vi "Get Item Reference By PathName.vi"(8 "error in (no error)":errorcluster, 10 "Item PathName":string, 11 "Root Item Reference in":T1 format="%.0x") -> (0 "error out":errorcluster, 2 "Item Reference":u64 format="%.0x", 3 "Root Item Reference out":T1 format="%.0x", 4 "found":bool)   [LabVIEW 2013, in "Hierarchy Framework.lvlib" / "Item.lvclass"]
uses:
  Item.lvclass
  Ctls/Item Reference.ctl
  Section/Section.lvclass
  Generic/Generic.lvclass
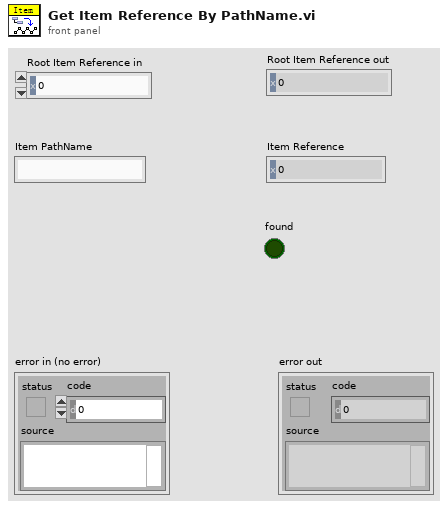
[diagram p1: front panel]
types:
  T1 = typedef "Hierarchy Framework.lvlib/Item.lvclass/Item Reference.ctl" = u64
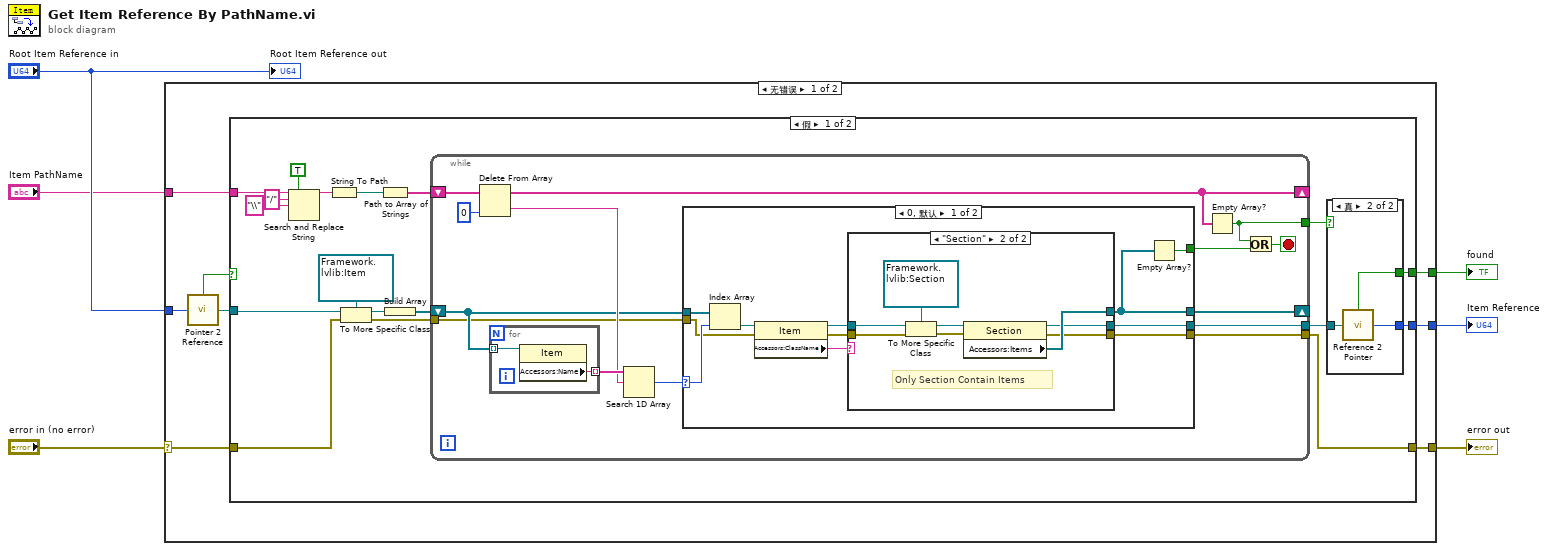
[diagram p0: block diagram]
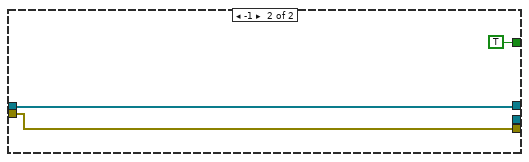
[diagram p4: hidden frame]
diagram:
  n1 = case shown="无错误" "error in (no error)" {
    selector: "error in (no error)" -> [w13 w77]
    tunnel: "Root Item Reference in" -> [w12 _]
    tunnel: [w14 w77] -> w5
    tunnel: [w9 _] -> w3
    tunnel: "Item PathName" -> [w8 _]
    tunnel: [w7 _] -> w1
    frame No Error {
      n2 = call "Pointer 2 Reference.vi"("Pointer"=w12) -> ("Not A Refnum?"=w11:bool, "Generic Reference"=w10:refnum<data-value>)
      n3 = case shown="假" w11 {
        tunnel: w13 -> [w31 w76]
        tunnel: [w25 w76] -> w14
        tunnel: w10 -> [w32 _]
        tunnel: [w16 _] -> w9
        tunnel: w8 -> [w22 _]
        tunnel: [w24 _] -> w7
        frame False {
          n4 = Search and Replace String(replace all?=TRUE ("替换全部？(F)"), input string=w22, search string="/" ("搜索字符串"), replace string="\\" ("替换字符串(\"\")")) -> (result string=w21:string)  [unwired: 4 in, 3 out]
          n5 = String To Path(string=w21) -> (path=w23:path)
          n6 = To More Specific Class(target class=refnum<data-value> refnum ("Item"), reference=w32, error in=w31) -> (specific class reference=w27:refnum<data-value>, error out=w26:errorcluster)
          n7 = Path to Array of Strings(0:w23) -> (2:w28:string[])  [unwired: 1 out]
          n8 = Build Array(w27) -> (w29:refnum<data-value>[])
          n9 = while {
            shift-right: [w45] -> _
            shift-left: w28 -> [w49]
            shift-right: [w41] -> _
            shift-left: w29 -> [w42]
            tunnel: [w40] -> w17
            tunnel: [w39] -> w25
            tunnel: w26 -> [w38]
            tunnel: [w36] -> w15
            stop <- w44 stop-if-true
            n10 = Delete From Array(array=w49, index=0 ("索引")) -> (deleted portion=w46:string, array with subset deleted=w45:string[])  [unwired: 1 in]
            n11 = for {
              tunnel: w42 -> [w75] mode=indexing
              tunnel: [w74] -> w47 mode=indexing
              n12 = property class="Item"(reference=w75) -> ("Accessors:Name"=w74:string)  [unwired: 1 in, 2 out]
            }
            n13 = Search 1D Array(1D array=w47, element=w46) -> (index of element=w43:i32)  [unwired: 1 in]
            n14 = case shown="0, 默认" w43 {
              selector: w43 -> [w59 _]
              tunnel: w42 -> [w60 w73]
              tunnel: [w50 w73] -> w41
              tunnel: [w54 _] -> w40
              tunnel: [w53 w72] -> w39
              tunnel: w38 -> [w52 w72]
              tunnel: [w51 TRUE] -> w37
              frame 0, Default {
                n15 = Index Array(array=w60, index=w59) -> (element=w58:refnum<data-value>)
                n16 = property class="Item"(reference=w58, error in=w52) -> (reference out=w56:refnum<data-value>, error out=w55:errorcluster, "Accessors:ClassName"=w57:string)
                n17 = case shown="\"Section\"" w57 {
                  tunnel: w56 -> [w62 w70]
                  tunnel: w55 -> [w61 w68]
                  tunnel: [_ w65] -> w50
                  tunnel: [w62 w64] -> w54
                  tunnel: [w61 w63] -> w53
                  frame "假", Default {
                  }
                  frame "Section" {
                    # "Only Section Contain Items"
                    n18 = To More Specific Class(target class=refnum<data-value> refnum ("Item"), reference=w70, error in=w68) -> (specific class reference=w67:refnum<data-value>, error out=w66:errorcluster)
                    n19 = property class="Section"(reference=w67, error in=w66) -> (reference out=w64:refnum<data-value>, error out=w63:errorcluster, "Accessors:Items"=w65:refnum<data-value>[])
                  }
                }
                n20 = Empty Array?(array=w50) -> (empty?=w51:bool)
              }
              frame -1 {
              }
            }
            n21 = Empty Array?(array=w45) -> (empty?=w36:bool)
            n22 = Or(x=w36, y=w37) -> (x .or. y?=w44:bool)
          }
          n23 = case shown="真" w15 {
            tunnel: [_ w35] -> w24
            tunnel: w17 -> [_ w34]
            tunnel: [_ w33] -> w16
            frame False {
            }
            frame True {
              n24 = call "Reference 2 Pointer.vi"("Generic Reference"=w34) -> ("Valid?"=w33:bool, "Pointer"=w35:u64)
            }
          }
        }
        frame True {
        }
      }
    }
    frame Error {
    }
  }
  "error out" <- w5
  "found" <- w3
  "Item Reference" <- w1
  "Root Item Reference out" <- "Root Item Reference in"
